vi "VolumeAndPressureRatioSamples.vi"() -> ()   [LabVIEW 2013]
panel:
  in  "VolumeAndPressureRatioSamples":cluster{"PressureRatios":dbl[], "Volumes":dbl[]}
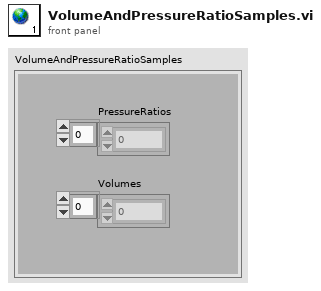
[diagram p1: front panel]
diagram:
